vi "Spartan HTTP Server Globals.vi"() -> ()   [LabVIEW 2011]
uses:
  Addons/internet/utils/keyedarr.llb/Keyed Array.ctl
  Spartan HTTP Session.ctl
  Addons/internet/http/http_obj.llb/HTTP Session Data.ctl
panel:
  in  "datasheet gen VI Refnum":refnum<vi>
  out "Reset Semaphore":bool
  out "TDM IO Lock Name":string
  out "num requests Lock":T1
  in  "CGI Refs":T2(array[cluster])
  out "LOG EVENT":refnum<user-event>
  in  "LOG_Q":refnum<queue>
  in  "HTTP_Q":refnum<queue>
  in  "num requests":u32
  out "server env":T3
  out "stop":bool
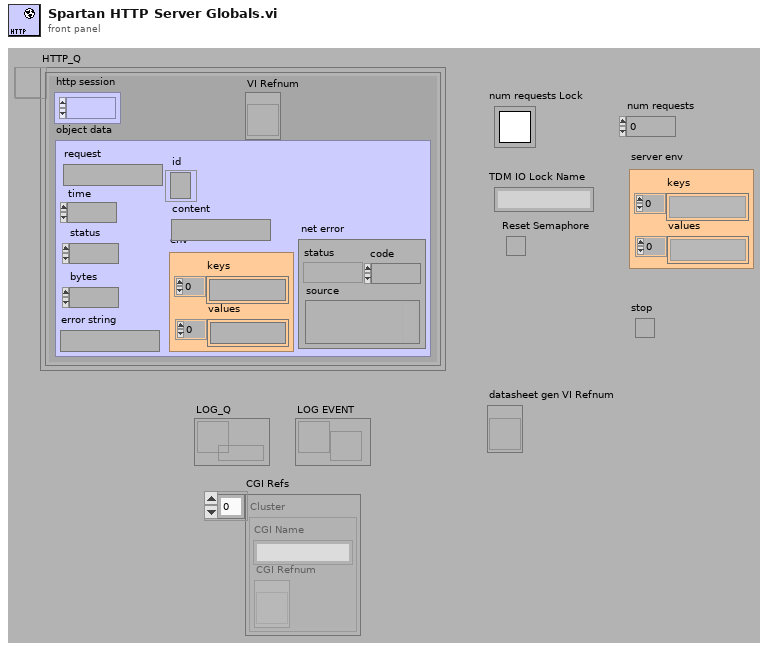
[diagram p1: front panel]
types:
  T1 = typedef "Semaphore RefNum" = refnum<k1>
  T2 = cluster{"CGI Name":string, "CGI Refnum":refnum<vi>}[]
  T3 = typedef "Keyed Array.ctl" = cluster{"keys":string[], "values":string[]}
diagram:
